vi "Write Selected images.vi"(8 "error in (no error)":errorcluster, 10 "Selected images":i32[](array[numeric]), 11 "HIS in":refnum<class "HIS.lvclass">) -> (0 "error out":errorcluster, 3 "HIS out":refnum<class "HIS.lvclass">)   [LabVIEW 2015, in "HIS.lvclass"]
uses:
  HIS.lvclass
  HIS.lvclass/HIS.ctl
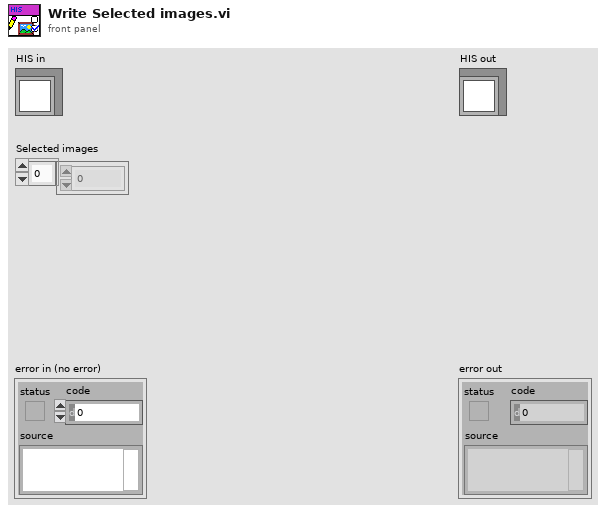
[diagram p1: front panel]
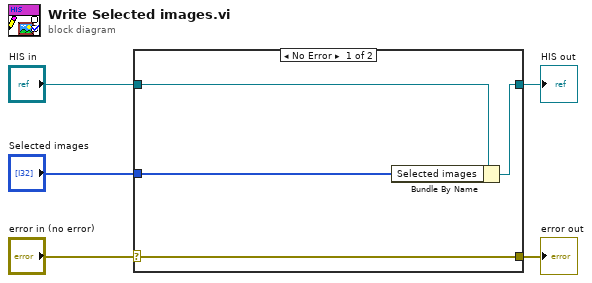
[diagram p0: block diagram]
diagram:
  n1 = case shown="No Error" "error in (no error)" {
    selector: "error in (no error)" -> [w9 w10]
    tunnel: [w9 w10] -> w4
    tunnel: [w7 w11] -> w2
    tunnel: "HIS in" -> [w8 w11]
    tunnel: "Selected images" -> [w6 _]
    frame No Error {
      n2 = Bundle By Name(cluster=w8, "Selected images"=w6) -> (w7:refnum<class "HIS.lvclass">)
    }
    frame Error {
    }
  }
  "error out" <- w4
  "HIS out" <- w2
